vi "TRIG_DEL.vi"(0 "VISA IN":refnum<visa-resource-name>, 5 "error in":errorcluster, 7 "Delay":dbl) -> (14 "VISA Out":refnum<visa-resource-name>, 19 "error out":errorcluster)   [LabVIEW 2018, in "PNA-X.lvlib"]
doc: "TRIGger:DELay <num> \n(Read-Write) Sets and reads the trigger delay. This delay is only applied while in External Trigger \nmode. After an external trigger is applied, the start of the sweep is held off for an amount of time \nequal to the delay setting plus any inherent latency. \nParameters \n<num> Delay value in seconds. Choose from 0 to 107. \nExamples TRIG:DEL .0003 \nSets the trigger delay to 300 microseconds. The sweep will not \nstart until approximately 300 microseconds after an external \ntrigger is applied. \nQuery Syntax TRIGger:DELay? \nReturn Type Numeric \nDefault 0 \n1893"
uses:
  PNA-X.lvlib
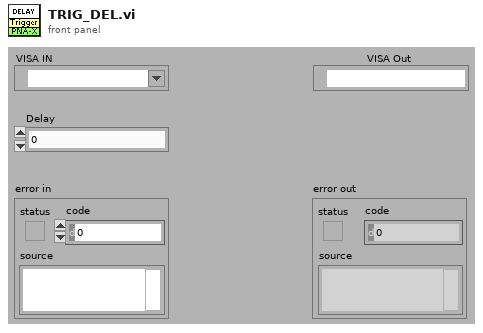
[diagram p1: front panel]
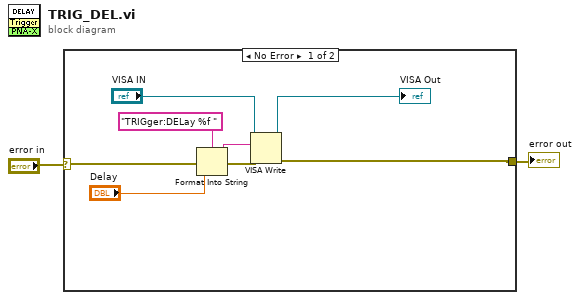
[diagram p0: block diagram]
diagram:
  n1 = case shown="No Error" "error in" {
    selector: "error in" -> [w10 w11]
    tunnel: [w5 w11] -> w1
    frame No Error {
      n2 = Format Into String(format string="TRIGger:DELay %f " ("Cmdline"), error in=w10, "Delay") -> (resulting string=w8:string, error out=w9:errorcluster)  [unwired: 1 in]
      n3 = VISA Write(VISA resource name="VISA IN", write buffer=w8, error in (no error)=w9) -> (VISA resource name out=→"VISA Out":refnum<visa-resource-name>, error out=w5:errorcluster)  [unwired: 1 out]
    }
    frame Error {
    }
  }
  "error out" <- w1
